vi "init.vi"(8 "error in":errorcluster, 10 "TBM module configuration in":refnum<class "TBM module configuration.lvclass">, 11 "Profibus Module runtime in":refnum<class "Profibus Module runtime.lvclass">) -> (0 "error out":errorcluster, 1 "data allocations":T1, 2 "execution settings":T4, 3 "Profibus Module runtime out":refnum<class "Profibus Module runtime.lvclass">)   [LabVIEW 2013, in "Profibus Module runtime.lvclass"]
doc: "Provides an interface for initializing a module at runtime. While this interface performs no operations, a child should provide an override which may open any necessary references or sessions, allocate necessary memory, and perform any final configuration validataion before providing the full configuration <b>execution data</b> to the calling process."
uses:
  Profibus Module runtime.lvclass
  <vilib>/NI/Tag Bus Module Framework/channel/TBM channel.lvclass
  <vilib>/NI/Tag Bus Module Framework/runtime/TBM module execution interface.lvclass
  configuration/Profibus Module configuration.lvclass
  <vilib>/rvi/interface/nirviOpenFPGA/nirviOpenFPGA.xnode
  <vilib>/rvi/interface/nirviMethod/nirviMethod.xnode
  <vilib>/addons/Comsoft.lib/cRIO PBMS/CS_cRIO-PB_DP-Master_FPGA-Reference.ctl
  <vilib>/FPGAPlugInAG/Dynamic/niLvFpga_Reset_Dynamic.vi
  <vilib>/FPGAPlugInAG/Dynamic/niLvFpga_Run_Dynamic.vi
  FPGA Bitfiles/ProfibusModule_FPGATarget_FPGAMain_wBXgaVGuACQ.lvbitx
  FPGA Main.vi
  <vilib>/FPGAPlugInAG/cRIO-9068/niLvFpga_Open_cRIO-9068.vi
  <vilib>/rvi/interface/common/dynamic/niFpgaDynamicAddResources.vi
  <vilib>/NI/Tag Bus Module Framework/module configuration/TBM module configuration.lvclass
  <vilib>/NI/Tag Bus Module Framework/runtime/execution settings.ctl
  <vilib>/NI/Tag Bus Module Framework/channel/data tables.ctl
  <vilib>/NI/Tag Bus/dictionary/data dictionary.lvclass
  <vilib>/NI/Tag Bus/dictionary table pair.ctl
  <vilib>/NI/Tag Bus/tag bus.lvlib
  <vilib>/NI/Tag Bus/table/data table.ctl
  <vilib>/NI/Tag Bus/table/data table.lvlib
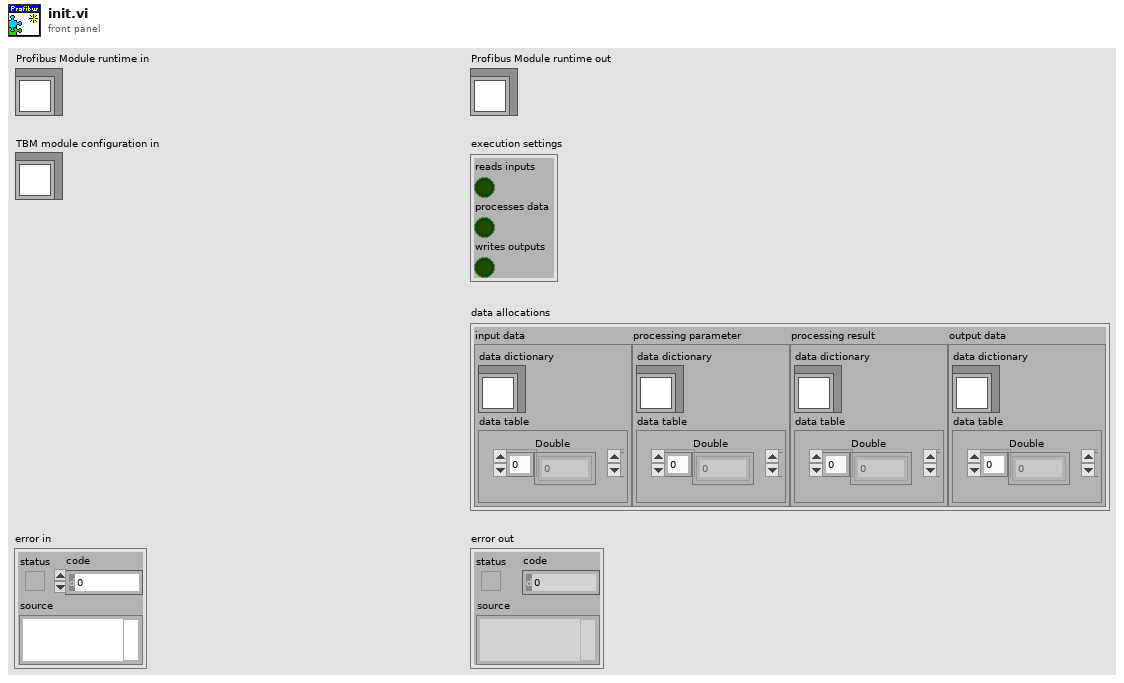
[diagram p1: front panel]
types:
  T1 = typedef "TBM channel.lvclass/data tables.ctl" = cluster{"input data":T2, "processing parameter":T2, "processing result":T2, "output data":T2}
  T2 = typedef "tag bus.lvlib/dictionary table pair.ctl" = cluster{"data dictionary":refnum<class "data dictionary.lvclass">, "data table":T3}
  T3 = typedef "tag bus.lvlib/data table.lvlib/data table.ctl" = cluster{"Double":dbl[], "Single":sgl[], "I64":i64[], "I32":i32[], "I16":i16[], "I8":i8[], "U64":u64[], "U32":u32[], "U16":u16[], "U8":u8[], "Boolean":bool[], "String":string[], "Array of Double":cluster{"DBL Array":dbl[]}[], "Array of Single":cluster{"SGL Array":sgl[]}[], "Array of I64":cluster{"I64 Array":i64[]}[], "Array of I32":cluster{"I32 Array":i32[]}[], "Array of I16":cluster{"I16 Array":i16[]}[], "Array of I8":cluster{"I8 Array":i8[]}[], "Array of U64":cluster{"U64 Array":u64[]}[], "Array of U32":cluster{"U32 Array":u32[]}[], "Array of U16":cluster{"U16 Array":u16[]}[], "Array of U8":cluster{"U8 Array":u8[]}[], "Array of Boolean":cluster{"Boolean Array":bool[]}[], "Array of String":cluster{"String Array":string[]}[]}
  T4 = typedef "TBM module execution interface.lvclass/execution settings.ctl" = cluster{"reads inputs":bool, "processes data":bool, "writes outputs":bool}
  T5 = typedef "CS_cRIO-PB_DP-Master_FPGA-Reference.ctl" = refnum<k20>
  T6 = cluster{"Address":i8, "Input Length":u8, "Output Length":u8}[]
  T7 = typedef "Profibus Module runtime.lvclass/profibus slave configuration.ctl" = cluster{"slave index":i8, "data items":T8[], "data buffer":u8[]}
  T8 = typedef "Profibus Module runtime.lvclass/profibus mapping configuration.ctl" = cluster{"data type":T9, " byte":i32, " bit":i32, "tag index":i32}
  T9 = typedef "tag bus.lvlib/tag descriptor.lvclass/Data Type.ctl" = enum16{"Double", "Single", "I64", "I32", "I16", "I8", "U64", "U32", "U16", "U8", "Boolean", "String", "Array of Double", "Array of Single", "Array of I64", "Array of I32", "Array of I16", "Array of I8", "Array of U64", "Array of U32", "Array of U16", "Array of U8", "Array of Boolean", "Array of String"}
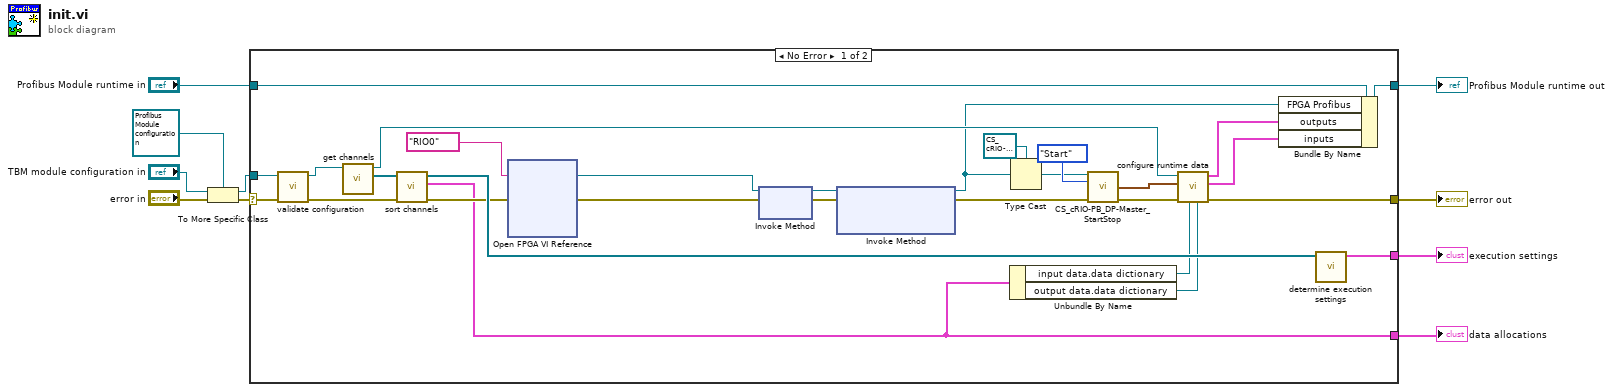
[diagram p0: block diagram]
diagram:
  n1 = To More Specific Class(target class=refnum<class "Profibus Module configuration.lvclass"> refnum ("Synchronous module configuration"), reference="TBM module configuration in", error in="error in") -> (specific class reference=w9:refnum<class "Profibus Module configuration.lvclass">, error out=w10:errorcluster)
  n2 = case shown="No Error" w10 {
    selector: w10 -> [w35 w40]
    tunnel: w9 -> [w34 _]
    tunnel: "Profibus Module runtime in" -> [w39 w41]
    tunnel: [w29 w41] -> w4
    tunnel: [w19 w40] -> w3
    tunnel: [w16 _] -> w1
    tunnel: [w38 _] -> w2
    frame No Error {
      n3 = call-dynamic "validate configuration.vi"("error in"=w35, "Profibus Module configuration in"=w34) -> ("error out"=w36:errorcluster, "Profibus Module configuration out"=w33:refnum<class "Profibus Module configuration.lvclass">)  [unwired: 8 in]
      n4 = call-dynamic "get channels.vi"("Profibus Module configuration in"=w33) -> ("channels"=w32:refnum<class "TBM channel.lvclass">[], "Profibus Module configuration out"=w17:refnum<class "Profibus Module configuration.lvclass">)  [unwired: 9 in]
      n5 = call <vilib>:"sort channels.vi"("error in"=w36, "channels in"=w32) -> ("error out"=w31:errorcluster, "data allocations"=w16:T1, "channels out"=w37:refnum<class "TBM channel.lvclass">[])  [unwired: 7 in]
      n6 = xnode "Open FPGA VI Reference"("error in"=w31, "resource name"=tag "RIO0") -> ("FPGA VI Reference Out"=w26:refnum<k20>, "error out"=w27:errorcluster)
      n7 = xnode "Invoke Method"("FPGA VI Reference In"=w26, "error in"=w27) -> ("FPGA VI Reference Out"=w25:refnum<k20>, "error out"=w28:errorcluster)
      n8 = xnode "Invoke Method"("FPGA VI Reference In"=w25, "error in"=w28) -> ("FPGA VI Reference Out"=w11:refnum<k20>, "error out"=w23:errorcluster)  [unwired: 1 in]
      n9 = Unbundle By Name(w16) -> ("input data.data dictionary"=w14:refnum<class "data dictionary.lvclass">, "output data.data dictionary"=w15:refnum<class "data dictionary.lvclass">)
      n10 = Type Cast(type=T5 refnum ("FPGA VI Reference out"), x=w11) -> (*(type *) &x=w13:T5)
      n11 = call <vilib>:"CS_cRIO-PB_DP-Master_StartStop.vi"("FPGA VI Reference"=w13, "DP-Master"=enum16{"Start", "Stop"}."Start", "Error"=w23) -> ("Slave Info List"=w18:T6, "Error out"=w20:errorcluster)  [unwired: 10 in, 1 out]
      n12 = call "configure runtime data.vi"("output dictionary"=w15, "input dictionary"=w14, "error in"=w20, "Slave Info List"=w18, "Profibus Module configuration in"=w17) -> ("error out"=w19:errorcluster, "inputs"=w21:T7[], "outputs"=w22:T7[])  [unwired: 4 in]
      n13 = Bundle By Name(cluster=w39, "FPGA Profibus"=w11, "outputs"=w22, "inputs"=w21) -> (w29:refnum<class "Profibus Module runtime.lvclass">)
      n14 = call <vilib>:"determine execution settings.vi"("channels"=w37) -> ("execution settings"=w38:T4)  [unwired: 10 in]
    }
    frame Error {
    }
  }
  "error out" <- w3
  "Profibus Module runtime out" <- w4
  "execution settings" <- w2
  "data allocations" <- w1
